vi "Determine Search Types from Selection.vi"(8 "error in (no error)":errorcluster, 11 "Search in":refnum<class "Search.lvclass">) -> (0 "error out":errorcluster, 2 "Search Type Infos":T1[](array[typedef]), 3 "Search":refnum<class "Search.lvclass">)   [LabVIEW 2020, in "Better Search.lvlib" / "Search.lvclass"]
uses:
  Search/Search.lvclass
  Data Types/Search Type Info.ctl
  Data Types/Search Type.ctl
  Search/Get Selection List.vi
  <vilib>/Utility/Data Type/NI_Data Type.lvlib
  Better Search.lvlib
panel:
  out "ClassNames":string[](array[string])
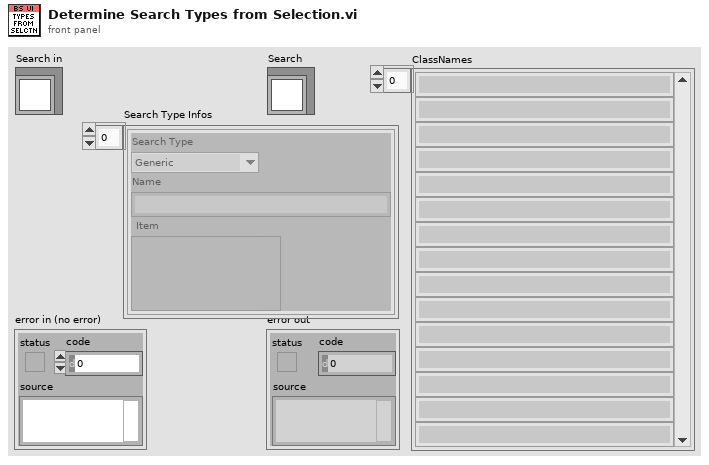
[diagram p1: front panel]
types:
  T1 = typedef "Better Search.lvlib/Search Type Info.ctl" = cluster{"Search Type":T2, "Name":string, "Item":variant}
  T2 = typedef "Better Search.lvlib/Search Type.ctl" = enum16{"Generic", "Text", "Data Type", "VI", "Node"}
  T3 = typedef "NI_Data Type.lvlib/Data Type.ctl" = enum8{"Invalid Type", "Void", "I8", "I16", "I32", "I64", "U8", "U16", "U32", "U64", "Single Float", "Double Float", "Extended Float", "Single Complex", "Double Complex", "Extended Complex", "Enum U8", "Enum U16", "Enum U32", "Enum U64", "Single Float With Unit", "Double Float With Unit", "Extended Float With Unit", "Single Complex with Unit", "Double Complex with Unit", "Extended Complex with Unit", "Boolean", "String", "Path", "Picture", "Tag", "Array", "Cluster", "Variant", "LV Variant", "Waveform", "Timestamp", "Digital Waveform", "Digital Data", "ExpressData", "Refnum", "External Data", "VI", "Poly VI", "LabVIEW Class Instance", "Fixed Point", "Set Collection", "Map Collection"}
  T4 = typedef "NI_Data Type.lvlib/Type Definition Info.ctl" = cluster{"Name":string, "Timestamp":u32}
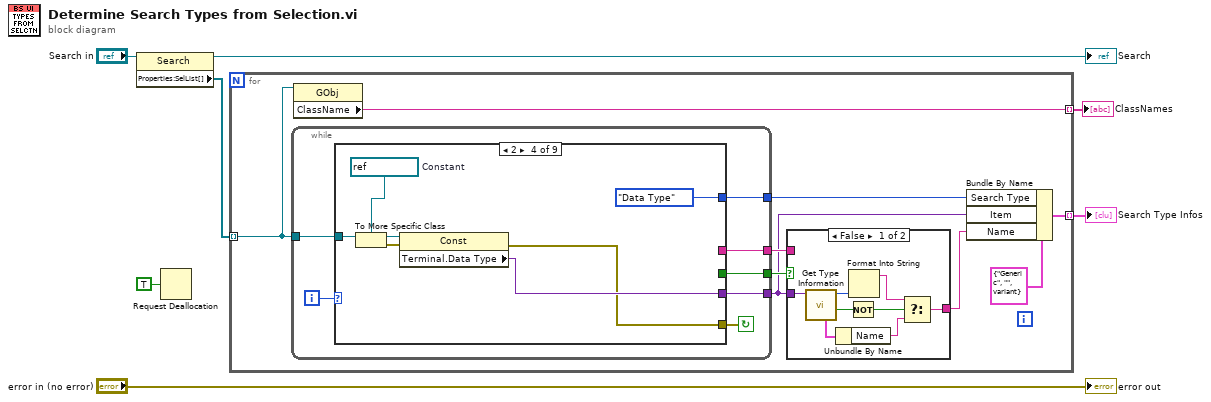
[diagram p0: block diagram]
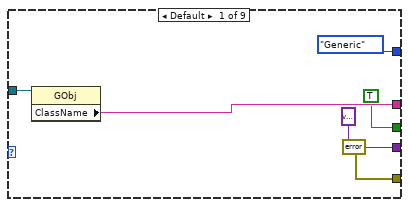
[diagram p2: hidden frame]
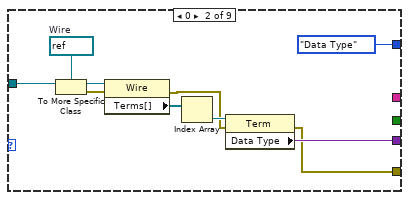
[diagram p3: hidden frame]
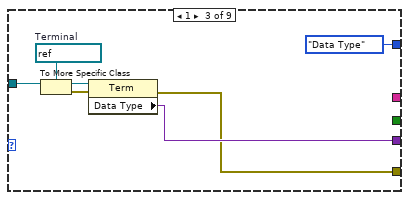
[diagram p4: hidden frame]
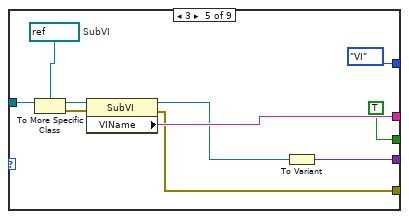
[diagram p5: hidden frame]
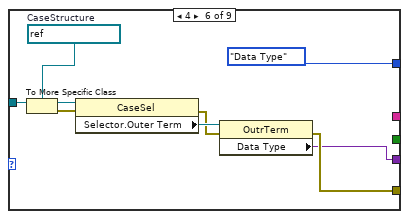
[diagram p6: hidden frame]
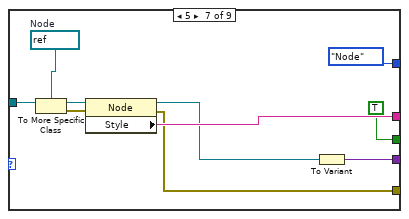
[diagram p7: hidden frame]
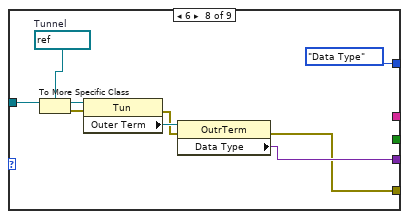
[diagram p8: hidden frame]
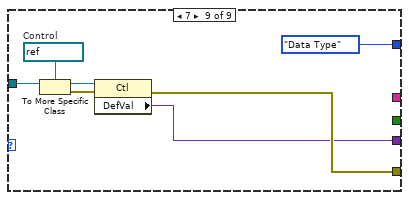
[diagram p9: hidden frame]
diagram:
  n1 = property class="Search"(reference="Search in") -> (reference out=→"Search":refnum<class "Search.lvclass">, "Properties:SelList[]"=w6:refnum<vi>[])  [unwired: 1 in, 1 out]
  n2 = Request Deallocation(TRUE ("flag")) -> ()
  n3 = for {
    tunnel: w6 -> [w9] mode=indexing
    tunnel: [w11] -> w4 mode=indexing
    tunnel: [w8] -> w2 mode=indexing
    n4 = while {
      tunnel: w9 -> [w23]
      tunnel: [w20] -> w10
      tunnel: [w19] -> w16
      tunnel: [w18] -> w15
      tunnel: [w17] -> w13
      i -> [w22]
      stop <- w21 continue-if-true
      n5 = case shown="2" w22 {
        tunnel: w23 -> [w29 w39 w46 w53 w63 w72 w82 w91 w98]
        tunnel: [errorcluster {"status"=FALSE, "code"=0, "source"=""} ("error out") w32 w42 w49 w58 w67 w77 w85 w93] -> w21
        tunnel: [variant ("Data Type") w35 w44 w51 w54 w66 w74 w88 w92] -> w20
        tunnel: [w28 _ _ _ w60 _ w80 _ _] -> w19
        tunnel: [TRUE _ _ _ TRUE _ TRUE _ _] -> w18
        tunnel: [Search_Type."Generic" ("Search Type") Search_Type."Data Type" ("Search Type") Search_Type."Data Type" ("Search Type") Search_Type."Data Type" ("Search Type") Search_Type."VI" ("Search Type") Search_Type."Data Type" ("Search Type") Search_Type."Node" ("Search Type") Search_Type."Data Type" ("Search Type") Search_Type."Data Type" ("Search Type")] -> w17
        frame Default {
          n6 = property class="GObj"(reference=w29) -> ("ClassName"=w28:string)  [unwired: 1 in, 2 out]
        }
        frame 0 {
          w31 = refnum<vi> refnum  # Wire
          n7 = To More Specific Class(target class=w31, reference=w39) -> (specific class reference=w38:refnum<vi>, error out=w34:errorcluster)  [unwired: 1 in]
          n8 = property class="Wire"(reference=w38, error in=w34) -> (error out=w33:errorcluster, "Terms[]"=w37:refnum<vi>[])  [unwired: 1 out]
          n9 = Index Array(array=w37) -> (element=w36:refnum<vi>)  [unwired: 1 in]
          n10 = property class="Term"(reference=w36, error in=w33) -> (error out=w32:errorcluster, "Data Type"=w35:variant)  [unwired: 1 out]
        }
        frame 1 {
          w41 = refnum<vi> refnum  # Terminal
          n11 = To More Specific Class(target class=w41, reference=w46) -> (specific class reference=w45:refnum<vi>, error out=w43:errorcluster)  [unwired: 1 in]
          n12 = property class="Term"(reference=w45, error in=w43) -> (error out=w42:errorcluster, "Data Type"=w44:variant)  [unwired: 1 out]
        }
        frame 2 {
          w48 = refnum<vi> refnum  # Constant
          n13 = To More Specific Class(target class=w48, reference=w53) -> (specific class reference=w52:refnum<vi>, error out=w50:errorcluster)  [unwired: 1 in]
          n14 = property class="Const"(reference=w52, error in=w50) -> (error out=w49:errorcluster, "Terminal.Data Type"=w51:variant)  [unwired: 1 out]
        }
        frame 3 {
          w57 = refnum<vi> refnum  # SubVI
          n15 = To More Specific Class(target class=w57, reference=w63) -> (specific class reference=w62:refnum<vi>, error out=w61:errorcluster)  [unwired: 1 in]
          n16 = property class="SubVI"(reference=w62, error in=w61) -> (reference out=w55:refnum<vi>, error out=w58:errorcluster, "VIName"=w60:string)
          n17 = To Variant(anything=w55) -> (Variant=w54:variant)
        }
        frame 4 {
          w65 = refnum<vi> refnum  # CaseStructure
          n18 = To More Specific Class(target class=w65, reference=w72) -> (specific class reference=w71:refnum<vi>, error out=w70:errorcluster)  [unwired: 1 in]
          n19 = property class="CaseSel"(reference=w71, error in=w70) -> (error out=w68:errorcluster, "Selector.Outer Term"=w69:refnum<vi>)  [unwired: 1 out]
          n20 = property class="OutrTerm"(reference=w69, error in=w68) -> (error out=w67:errorcluster, "Data Type"=w66:variant)  [unwired: 1 out]
        }
        frame 5 {
          w76 = refnum<vi> refnum  # Node
          n21 = To More Specific Class(target class=w76, reference=w82) -> (specific class reference=w81:refnum<vi>, error out=w78:errorcluster)  [unwired: 1 in]
          n22 = property class="Node"(reference=w81, error in=w78) -> (reference out=w73:refnum<vi>, error out=w77:errorcluster, "Style"=w80:string)
          n23 = To Variant(anything=w73) -> (Variant=w74:variant)
        }
        frame 6 {
          w84 = refnum<vi> refnum  # Tunnel
          n24 = To More Specific Class(target class=w84, reference=w91) -> (specific class reference=w90:refnum<vi>, error out=w87:errorcluster)  [unwired: 1 in]
          n25 = property class="Tun"(reference=w90, error in=w87) -> (error out=w86:errorcluster, "Outer Term"=w89:refnum<vi>)  [unwired: 1 out]
          n26 = property class="OutrTerm"(reference=w89, error in=w86) -> (error out=w85:errorcluster, "Data Type"=w88:variant)  [unwired: 1 out]
        }
        frame 7 {
          w95 = refnum<vi> refnum  # Control
          n27 = To More Specific Class(target class=w95, reference=w98) -> (specific class reference=w97:refnum<vi>, error out=w96:errorcluster)  [unwired: 1 in]
          n28 = property class="Ctl"(reference=w97, error in=w96) -> (error out=w93:errorcluster, "DefVal"=w92:variant)  [unwired: 1 out]
        }
      }
    }
    n29 = property class="GObj"(reference=w9) -> ("ClassName"=w8:string)  [unwired: 1 in, 2 out]
    n30 = case shown="False" w15 {
      tunnel: w16 -> [_ w107]
      tunnel: [w99 w107] -> w12
      tunnel: w10 -> [w106 _]
      frame False {
        n31 = call <vilib>:"Get Type Information.vi"("variant"=w106) -> ("type definition"=w104:bool, "type"=w105:T3, "type definition info"=w101:T4)  [unwired: 6 in, 2 out]
        n32 = Unbundle By Name(w101) -> ("Name"=w100:string)
        n33 = Not(x=w104) -> (.not. x?=w102:bool)
        n34 = Format Into String(w105) -> (resulting string=w103:string)  [unwired: 3 in, 1 out]
        n35 = Select(t=w103, s=w102, f=w100) -> (s? t:f=w99:string)
      }
      frame True {
      }
    }
    n36 = Bundle By Name(cluster=T1 {"Search Type"=enum."Generic", "Name"="", "Item"=variant(refnum<vi> refnum)} ("Search Type Info"), "Search Type"=w13, "Item"=w10, "Name"=w12) -> (w11:T1)
  }
  "Search Type Infos" <- w4
  "ClassNames" <- w2
  "error out" <- "error in (no error)"
